vi "Pt_Thermometer_IVcurves.vi"() -> ()   [LabVIEW 2016]
uses:
  Instance          10 31Saved   Pt_Thermometer_IVcurves .vi
  Instance           9 31Saved   Pt_Thermometer_IVcurves .vi
  Instance           8 31Saved   Pt_Thermometer_IVcurves .vi
  Instance           6 31Saved   Pt_Thermometer_IVcurves .vi
  Instance           5 31Saved   Pt_Thermometer_IVcurves .vi
  Instance           4 31Saved   Pt_Thermometer_IVcurves .vi
  <vilib>/Utility/file.llb/Write To Spreadsheet File (DBL).vi
  <vilib>/Utility/file.llb/Read From Spreadsheet File (DBL).vi
panel:
  out "V2ptB":dbl[](array[numeric])
  out "I2ptB":dbl[](array[numeric])
  in  "Temperature at which \nmeasurement is done (K)":string
  out "IV characteristic of Pt Thermometer B (COLD END)\nSMU 3 and 4":cluster{"Y":dbl[], "Y":dbl[]}[](graph)
  out "IV characteristic of Pt Thermometer A (HOT END) SMU 1 and 2":cluster{"Y":dbl[], "Y":dbl[]}[](graph)
  in  "File Path":path
  out "V2ptA":dbl[](array[numeric])
  out "I2ptA":dbl[](array[numeric])
  in  "Current through Pt Thermometers":T1
  out "error out":errorcluster
  in  "error in (no error)":errorcluster
  in  "4155C VISA resource name":refnum<visa-resource-name>
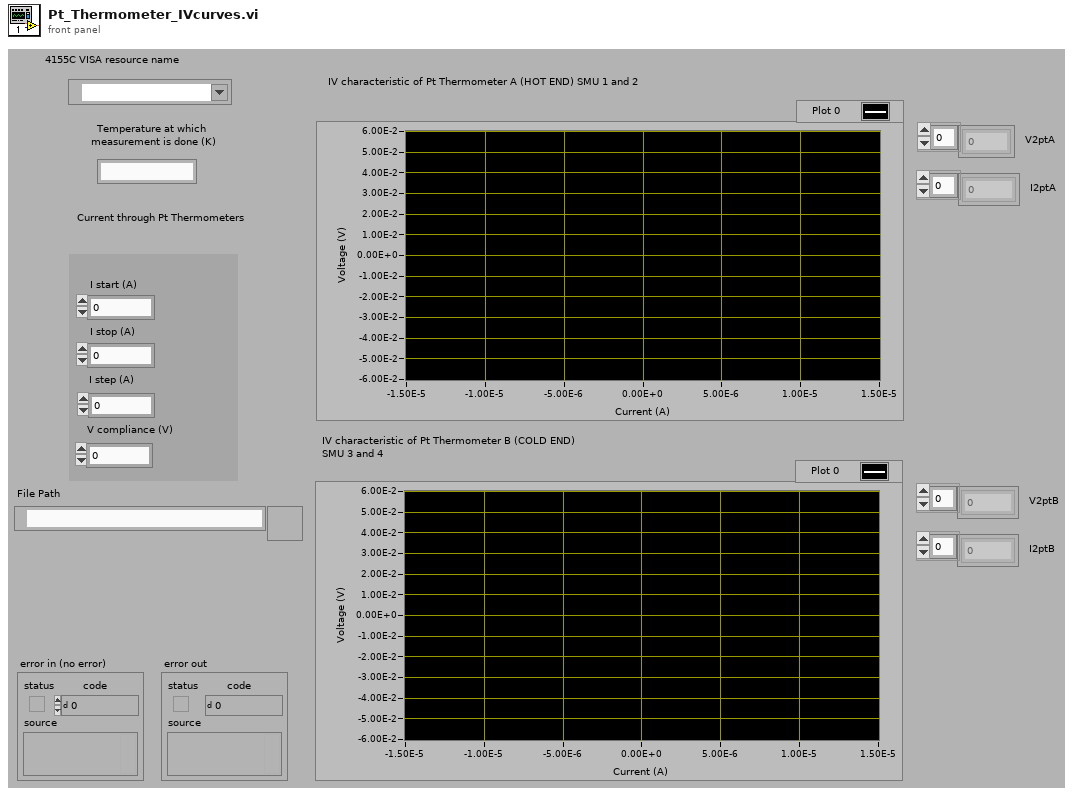
[diagram p1: front panel]
types:
  T1 = cluster{"I start (A)":dbl, "I stop (A)":dbl, "I step (A)":dbl, "V compliance (V)":dbl}
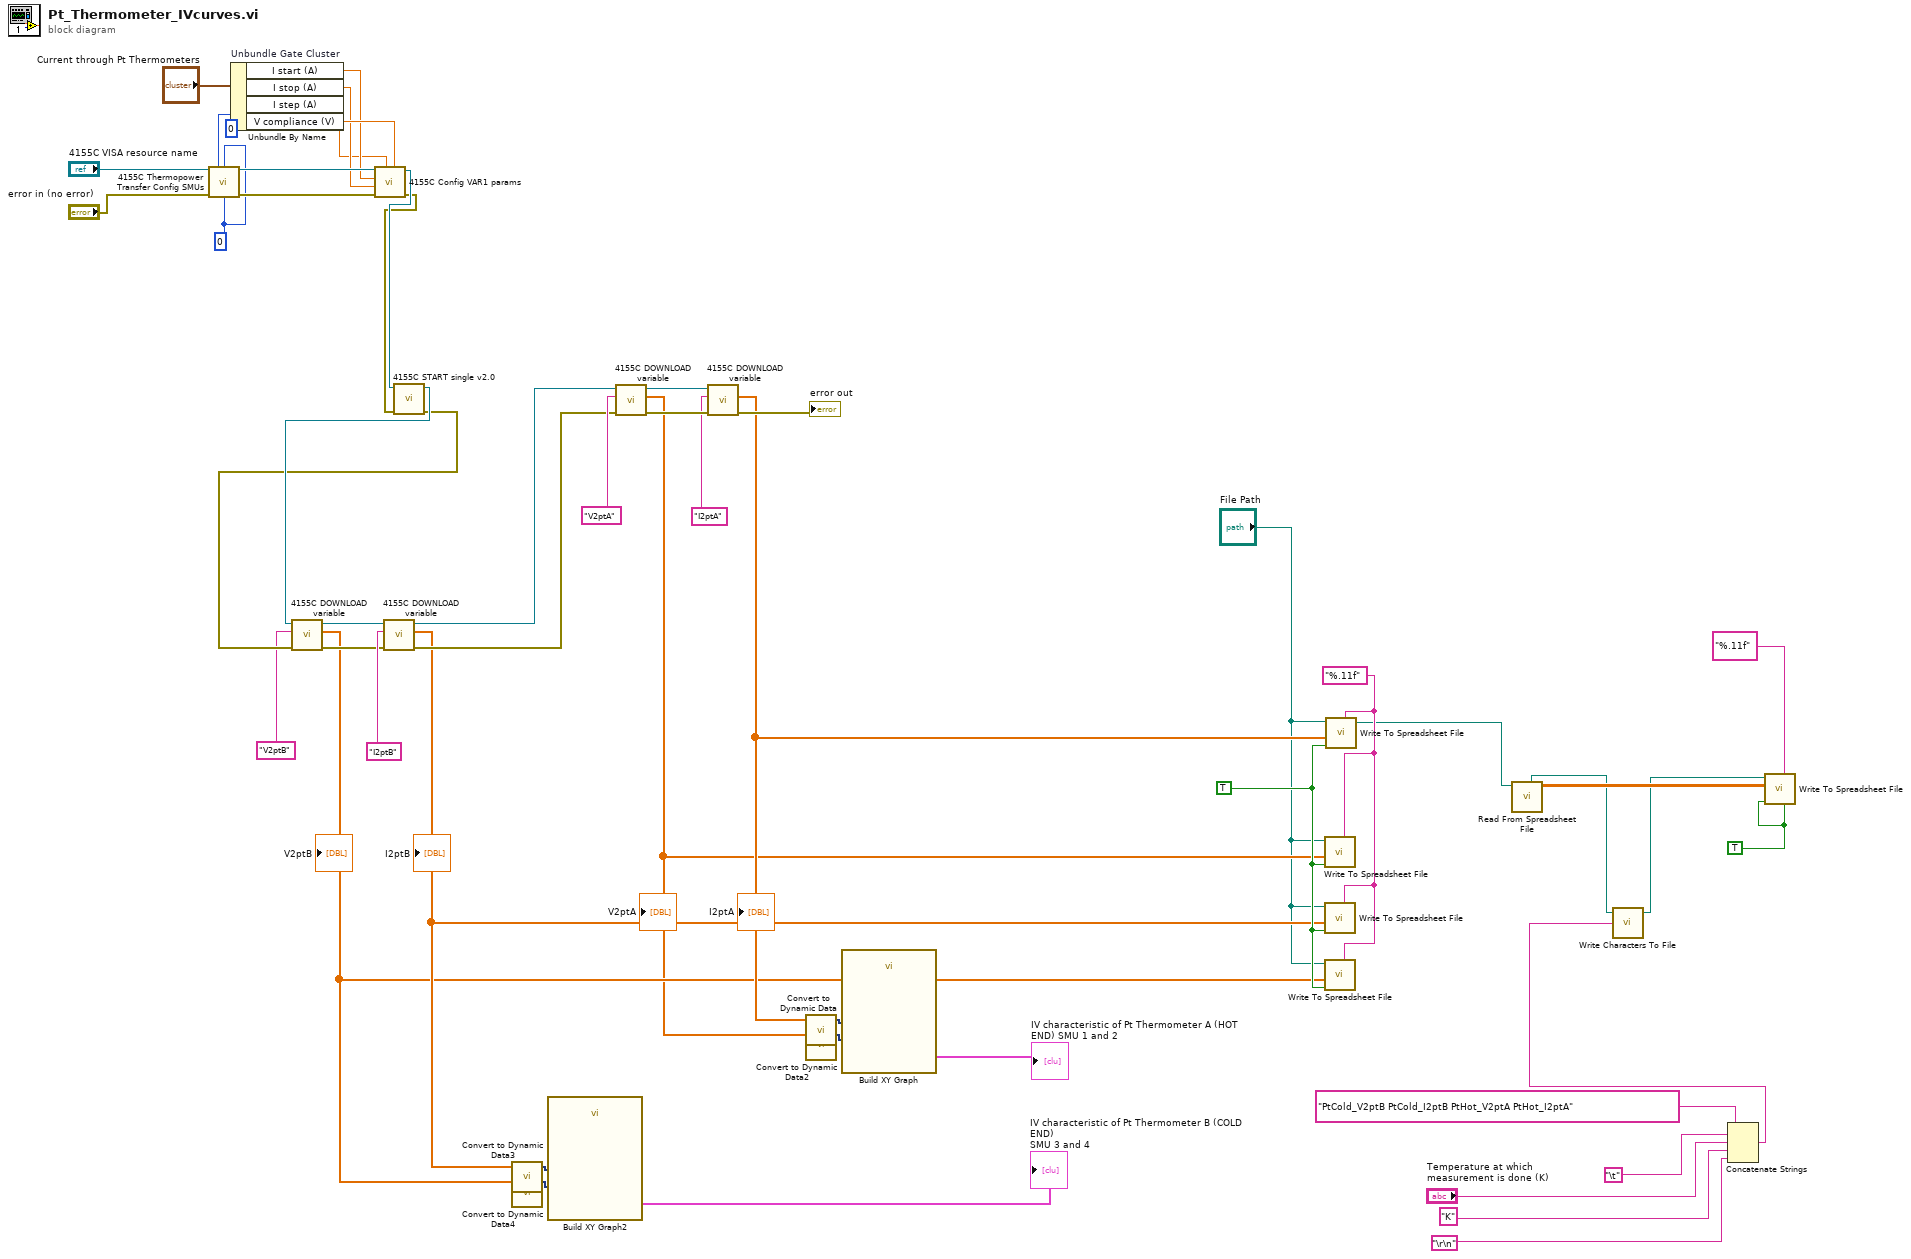
[diagram p0: block diagram]
diagram:
  w11 = TRUE
  w20 = "%.11f"
  w24 = TRUE
  w39 = 0
  n1 = call "4155C Thermopower Transfer Config SMUs.vi"("VISA resource name in"="4155C VISA resource name", "sweep method"=0, "Gate mode"=w39, "error in (no error)"="error in (no error)", "Source/drain mode"=w39) -> ("VISA Resource Name out"=w41:refnum<visa-resource-name>, "error out"=w42:errorcluster)  [unwired: 8 in, 1 out]
  n2 = Unbundle By Name "Unbundle Gate Cluster"("Current through Pt Thermometers") -> ("I start (A)"=w5:dbl, "I stop (A)"=w4:dbl, "I step (A)"=w3:dbl, "V compliance (V)"=w6:dbl)
  n3 = call "4155C Config VAR1 params.vi"("compliance"=w6, "step (linear only)"=w3, "error in (no error)"=w42, "stop"=w4, "start"=w5, "VISA session"=w41) -> ("error out"=w1:errorcluster, "dup VISA resource name"=w2:refnum<visa-resource-name>)  [unwired: 3 in, 1 out]
  n4 = call "4155C START single v2.0.vi"("error in (no error)"=w1, "VISA resource name in"=w2) -> ("error out"=w34:errorcluster, "VISA Resource Name out"=w35:refnum<visa-resource-name>)  [unwired: 1 in, 3 out]
  n5 = call "4155C DOWNLOAD variable.vi"("error in (no error)"=w34, "Variable name"="V2ptB", "VISA resource name in"=w35) -> ("error out"=w36:errorcluster, "Output data"=w22:dbl[], "VISA Resource Name out"=w37:refnum<visa-resource-name>)  [unwired: 2 out]
  "V2ptB" <- w22
  n6 = call "4155C DOWNLOAD variable.vi"("error in (no error)"=w36, "Variable name"="I2ptB", "VISA resource name in"=w37) -> ("error out"=w32:errorcluster, "Output data"=w23:dbl[], "VISA Resource Name out"=w33:refnum<visa-resource-name>)  [unwired: 2 out]
  "I2ptB" <- w23
  n7 = call "Convert to Dynamic Data3"("Array"=w23) -> ("Dynamic Data Type"=w31:dynamicdata)  [unwired: 3 out]
  n8 = call "Convert to Dynamic Data4"("Array"=w22) -> ("Dynamic Data Type"=w30:dynamicdata)  [unwired: 3 out]
  n9 = call "Build XY Graph2"("Y Input"=w30, "X Input"=w31) -> ("XY Graph"=→"IV characteristic of Pt Thermometer B (COLD END)\nSMU 3 and 4":cluster{"Y":dbl[], "Y":dbl[]}[])  [unwired: 3 in, 6 out]
  n10 = call "4155C DOWNLOAD variable.vi"("error in (no error)"=w32, "Variable name"="V2ptA", "VISA resource name in"=w33) -> ("error out"=w49:errorcluster, "Output data"=w21:dbl[], "VISA Resource Name out"=w50:refnum<visa-resource-name>)  [unwired: 2 out]
  "V2ptA" <- w21
  n11 = call "4155C DOWNLOAD variable.vi"("error in (no error)"=w49, "Variable name"="I2ptA", "VISA resource name in"=w50) -> ("error out"=→"error out":errorcluster, "Output data"=w25:dbl[])  [unwired: 3 out]
  "I2ptA" <- w25
  n12 = call "Convert to Dynamic Data"("Array"=w25) -> ("Dynamic Data Type"=w47:dynamicdata)  [unwired: 3 out]
  n13 = call "Convert to Dynamic Data2"("Array"=w21) -> ("Dynamic Data Type"=w46:dynamicdata)  [unwired: 3 out]
  n14 = call "Build XY Graph"("Y Input"=w46, "X Input"=w47) -> ("XY Graph"=→"IV characteristic of Pt Thermometer A (HOT END) SMU 1 and 2":cluster{"Y":dbl[], "Y":dbl[]}[])  [unwired: 3 in, 6 out]
  n15 = call-poly <vilib>:"Write To Spreadsheet File.vi"("format (%.3f)"=w20, "append to file? (new file:F)"=w24, "1D data"=w21, "file path (dialog if empty)"="File Path") -> ()  [unwired: 2 in, 3 out]
  n16 = call-poly <vilib>:"Write To Spreadsheet File.vi"("format (%.3f)"=w20, "append to file? (new file:F)"=w24, "1D data"=w23, "file path (dialog if empty)"="File Path") -> ()  [unwired: 2 in, 3 out]
  n17 = call-poly <vilib>:"Write To Spreadsheet File.vi"("format (%.3f)"=w20, "append to file? (new file:F)"=w24, "1D data"=w22, "file path (dialog if empty)"="File Path") -> ()  [unwired: 2 in, 3 out]
  n18 = call-poly <vilib>:"Write To Spreadsheet File.vi"("format (%.3f)"=w20, "append to file? (new file:F)"=w24, "1D data"=w25, "file path (dialog if empty)"="File Path") -> ("new file path (Not A Path if cancelled)"=w15:path)  [unwired: 2 in, 2 out]
  n19 = call-poly <vilib>:"Read From Spreadsheet File.vi"("file path (dialog if empty)"=w15) -> ("all rows"=w17:dbl[][], "new file path (Not A Path if cancelled)"=w14:path)  [unwired: 3 in, 6 out]
  n20 = Concatenate Strings("PtCold_V2ptB PtCold_I2ptB PtHot_V2ptA PtHot_I2ptA", "\t", "Temperature at which \nmeasurement is done (K)", "K", "\r\n") -> (w12:string)
  n21 = call <vilib>:"Write Characters To File.vi"("character string"=w12, "file path (dialog if empty)"=w14) -> ("new file path (Not A Path if cancelled)"=w13:path)  [unwired: 1 in, 2 out]
  n22 = call-poly <vilib>:"Write To Spreadsheet File.vi"("transpose? (no:F)"=w11, "format (%.3f)"="%.11f", "append to file? (new file:F)"=w11, "2D data"=w17, "file path (dialog if empty)"=w13) -> ()  [unwired: 1 in, 3 out]
